vi "Trap2-11-15.vi"(0 "Heizen?Trap2":bool, 2 "Per[us]Trap2":u32 caption="PerTrap2[us]", 5 "PIDTrap2":T1 {"proportional gain (Kc)" format="%.11g"; "integral gain (Kc*Ts/Ti)" format="%.11g"; "derivative gain (Kc*Td/Ts)" format="%.11g"}, 7 "UTempMaxTrap2":fxp<+/-,16,4> format="%.14g", 11 "UTempSPTrap2":fxp<+/-,16,4> format="%.14g", 13 "warten[us]Trap2":u32=200) -> (4 "UTemp[V]Trap2":fxp<+/-,16,4> format="%.25g")   [LabVIEW 2010]
uses:
  <vilib>/eio/EIONode/EIONode.xnode
  <vilib>/rvi/eio/nirviEIOImplementation/nirviEIOImplementation.xnode
  <vilib>/rvi/eio/common/nirviEmuClasses.ctl
  <vilib>/addons/control/pid/fpga.llb/XNode/niFpgaPID.xnode
  <vilib>/rvi/eio/common/nirviEmuTemplateMethod_noerrors.vi
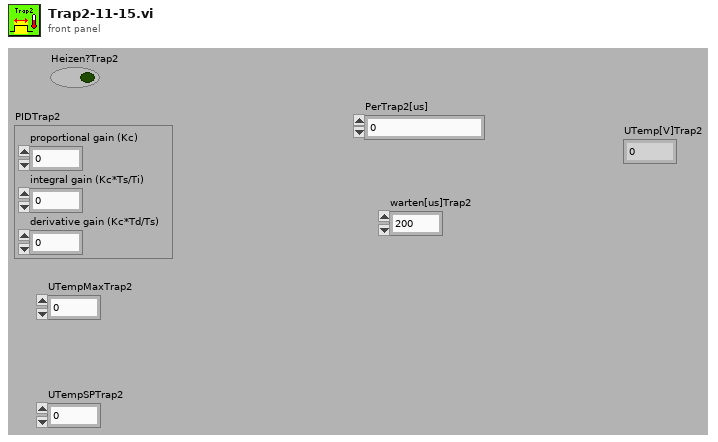
[diagram p1: front panel]
types:
  T1 = cluster{"proportional gain (Kc)":fxp<+/-,16,8>, "integral gain (Kc*Ts/Ti)":fxp<+/-,16,8>, "derivative gain (Kc*Td/Ts)":fxp<+/-,16,8>}
  T2 = cluster{"output high":fxp<+/-,16,4>, "output low":fxp<+/-,16,4>}
  T3 = typedef "nirviEmuClasses.ctl" = enum16{"IO Read", "IO Write", "Method", "Property Read", "Property Write"}
  T4 = cluster{"proportional gain (Kc)":i16, "integral gain (Kc*Ts/Ti)":i16, "derivative gain (Kc*Td/Ts)":i16}
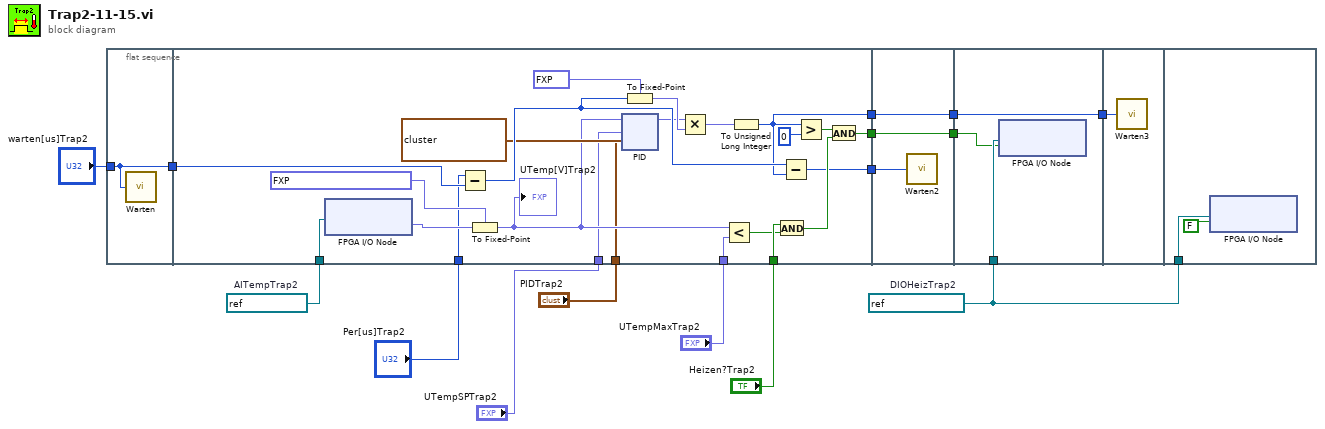
[diagram p0: block diagram]
diagram:
  w6 = refnum<k21> "Mod1/AI1"  # AITempTrap2
  w5 = refnum<k21> "Mod6/DIO18"  # DIOHeizTrap2
  n1 = flat-sequence {
    tunnel: [w16] -> w15
    tunnel: "warten[us]Trap2" -> [w16]
    tunnel: w6 -> [w39]
    tunnel: [w34] -> w14
    tunnel: w15 -> [w26]
    tunnel: [w32] -> w13
    tunnel: [w31] -> w12
    tunnel: "Per[us]Trap2" -> [w22]
    tunnel: "PIDTrap2" -> [w21]
    tunnel: "UTempMaxTrap2" -> [w20]
    tunnel: "Heizen?Trap2" -> [w19]
    tunnel: "UTempSPTrap2" -> [w18]
    tunnel: [w97] -> w11
    tunnel: w14 -> [w97]
    tunnel: [w96] -> w10
    tunnel: w13 -> [w96]
    tunnel: w12 -> [w95]
    tunnel: w5 -> [w100]
    tunnel: w11 -> [w99]
    tunnel: [w98] -> w9
    tunnel: w10 -> [w98]
    tunnel: w9 -> [w112]
    tunnel: w5 -> [w114]
    frame #0 {
      n2 = call "Warten"("Count(uSec)"=w16) -> ()  [unwired: 1 out]
    }
    frame #1 {
      n3 = xnode "FPGA I/O Node"("FPGA I/O In"=w39) -> ("I/O Item"=w24:fxp<+/-,26,5>)  [unwired: 1 out]
      n4 = Subtract(x=w22, y=w26) -> (x-y=w33:u32)
      n5 = To Fixed-Point(fixed-point type=fxp<+/-,16,4> 0.0 ("Festkommatyp"), number=w24) -> (fixed-point=w23:fxp<+/-,16,4>)
      "UTemp[V]Trap2" <- w23
      n6 = xnode ("PID")("process variable"=w23, "setpoint"=w18, "PID gains"=w21, "output range"=T2 {"output high"=1.0, "output low"=0.0}) -> ("output"=w27:fxp<+/-,16,4>)  [unwired: 1 in]
      n7 = To Fixed-Point(fixed-point type=fxp<+/-,21,21> 32768.0 ("output high"), number=w33) -> (fixed-point=w30:fxp<+/-,21,21>)
      n8 = Multiply(x=w27, y=w30) -> (x*y=w29:fxp<+/-,37,25>)
      n9 = Less?(x=w23, y=w20) -> (x < y?=w17:bool)
      n10 = To Unsigned Long Integer(number=w29) -> (unsigned 32bit integer=w32:u32)
      n11 = And(x=w19, y=w17) -> (x .and. y?=w35:bool)
      n12 = Subtract(x=w33, y=w32) -> (x-y=w31:u32)
      n13 = Greater?(x=w32, y=u32 0) -> (0:w36:bool)
      n14 = And(x=w36, y=w35) -> (x .and. y?=w34:bool)
    }
    frame #2 {
      n15 = call "Warten2"("Count(uSec)"=w95) -> ()  [unwired: 1 out]
    }
    frame #3 {
      n16 = xnode "FPGA I/O Node"("I/O Item"=w99, "FPGA I/O In"=w100) -> ()  [unwired: 1 out]
    }
    frame #4 {
      n17 = call "Warten3"("Count(uSec)"=w112) -> ()  [unwired: 1 out]
    }
    frame #5 {
      n18 = xnode "FPGA I/O Node"("I/O Item"=FALSE, "FPGA I/O In"=w114) -> ()  [unwired: 1 out]
    }
  }
